vi "joint.vi"() -> ()   [LabVIEW 2023]
panel:
  out "CH2_spreadsheet":string
  out "CH2_array_units":dbl[][](array[numeric])
  out "CH2_Time":dbl[](array[numeric])
  out "CH2_Voltage":dbl[](array[numeric])
  out "CH2_array":dbl[][](array[numeric])
  out "concatenated string 2":string
  out "CH2_file":string
  in  "match button":bool
  in  "STOP":bool
  in  "Export button":bool
  out "CH1_spreadsheet":string
  out "CH1_array_units":dbl[][](array[numeric])
  out "CH1_Time":dbl[](array[numeric])
  out "CH1_Voltage":dbl[](array[numeric])
  out "CH1_file":string
  in  "index":i32 min=0 max=20
  out "CH1_array":dbl[][](array[numeric])
  out "concatenated string":string
  in  "R (Ω)":string
  in  "Current mode":bool
  in  "Extract button":bool
  out "standard output":string
  in  "CH2_units":string(combo)
  in  "∆V CH2":string
  in  "CH1_units":string(combo)
  in  "∆V CH1":string
  in  "t units":string(combo)
  in  "∆t":string
  out "CH1":bool
  out "CH2":bool
  in  "Select channel":bool
  in  "Output path":path
  in  "Input path":path
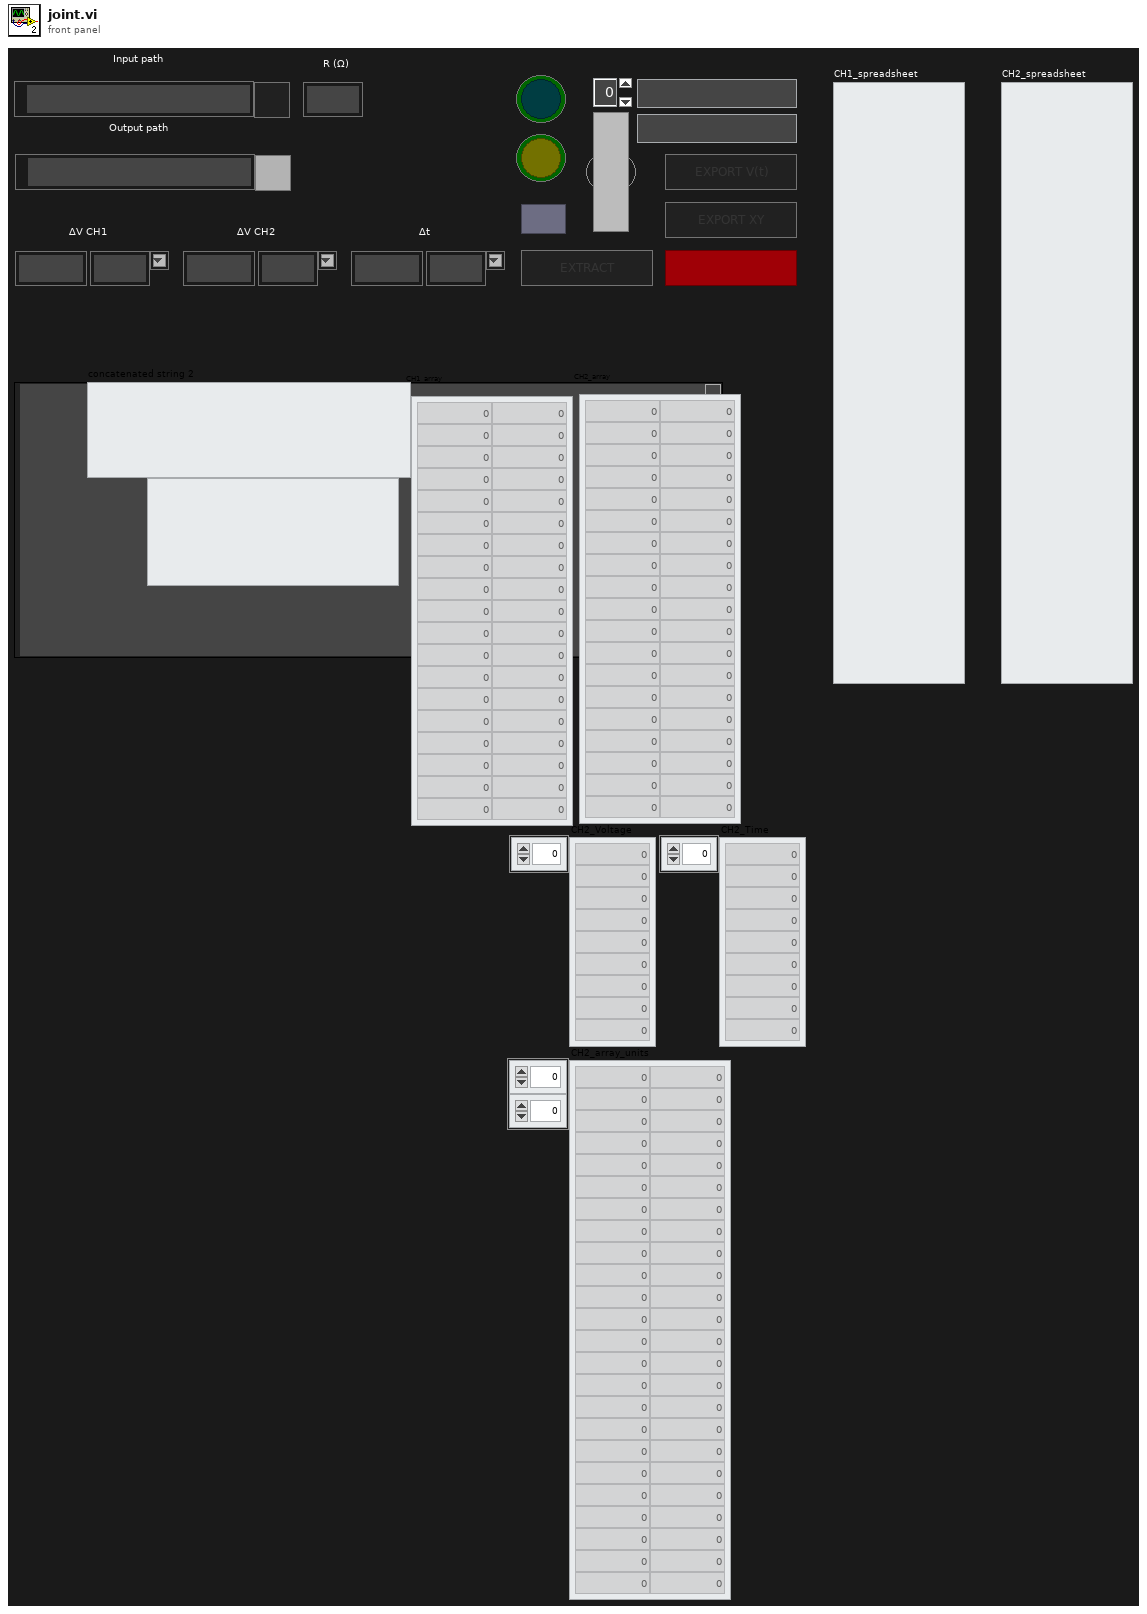
[diagram p1: front panel]
types:
  T1 = enum16{"open", "replace", "create", "open or create", "replace or create", "replace or create with confirmation"}
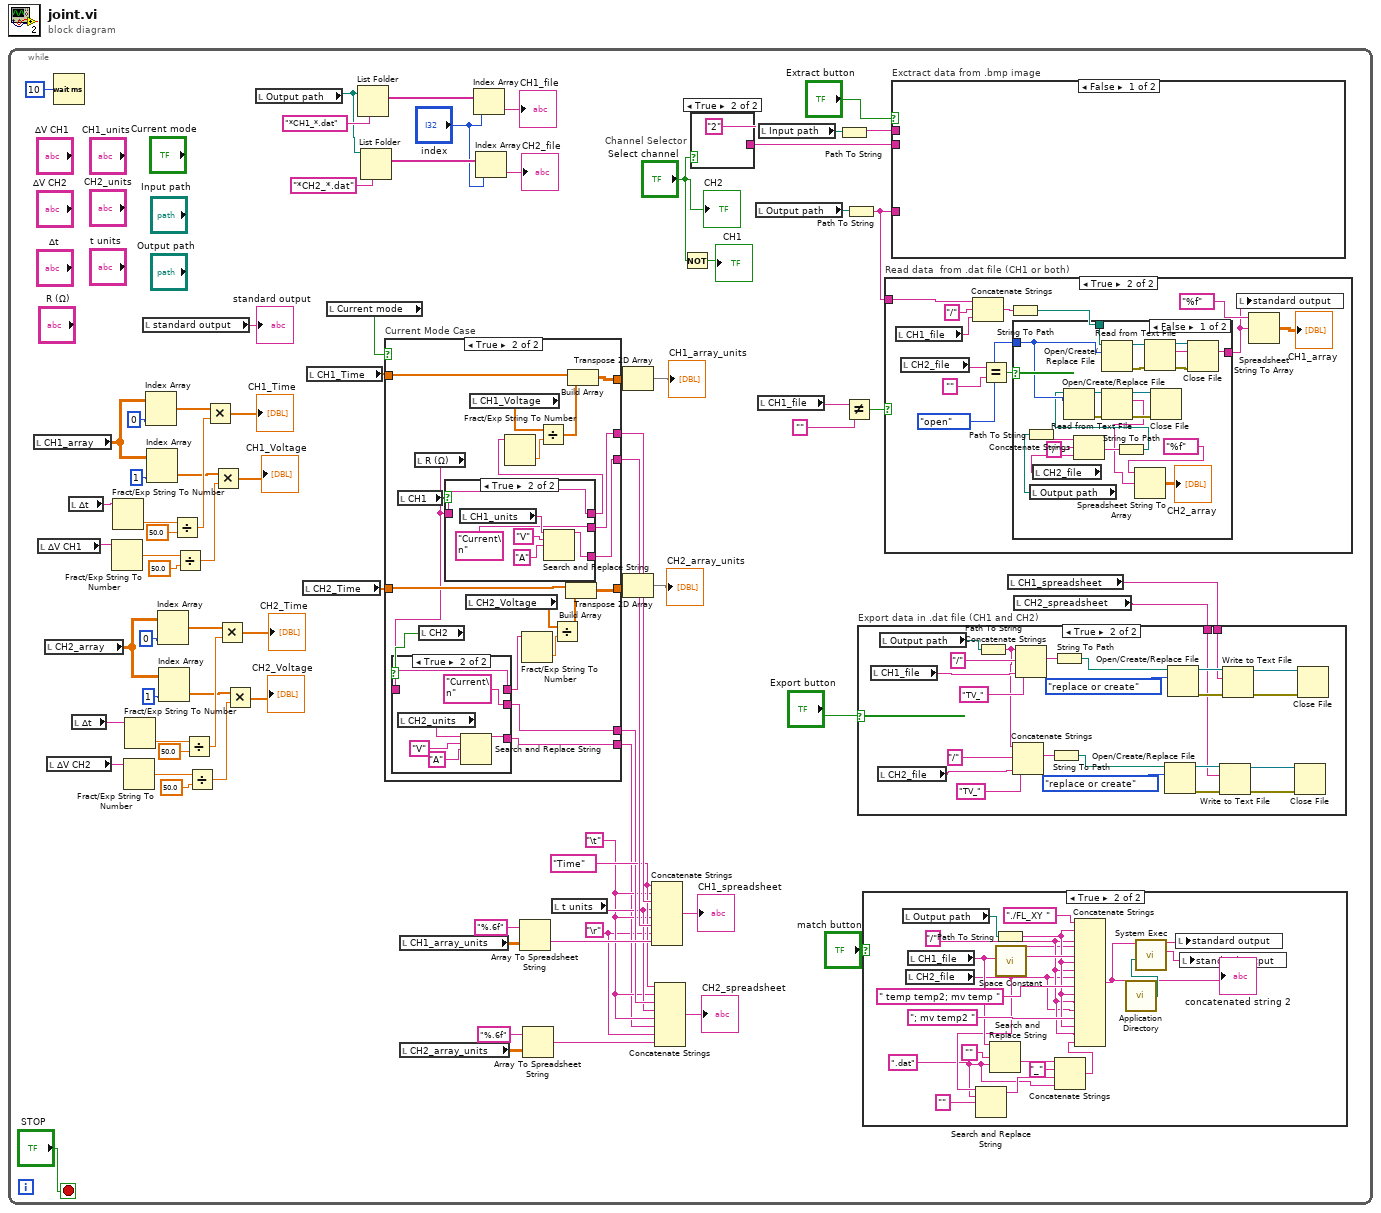
[diagram p0: block diagram]
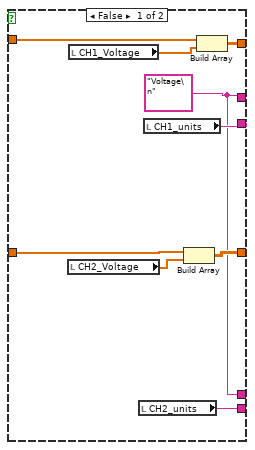
[diagram p2: hidden frame]
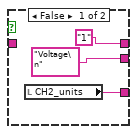
[diagram p3: hidden frame]
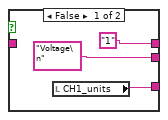
[diagram p4: hidden frame]
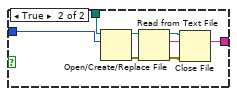
[diagram p8: hidden frame]
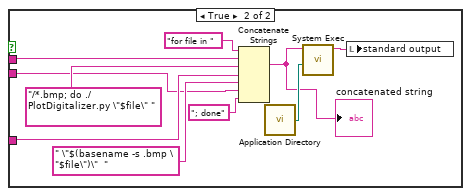
[diagram p9: hidden frame]
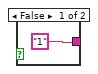
[diagram p10: hidden frame]
diagram:
  n1 = while {
    stop <- "STOP" stop-if-true
    w4 = "\r"
    w6 = "\t"
    w9 = "Time" ("string")
    n2 = local read "CH1_array"() -> (w72:dbl[][])
    n3 = local read "∆V CH1"() -> (w41:string)
    n4 = local read "CH2_array"() -> (w25:dbl[][])
    n5 = local read "∆V CH2"() -> (w23:string)
    n6 = Wait (ms)(milliseconds to wait=u32 10) -> ()  [unwired: 1 out]
    n7 = local read "∆t"() -> (w65:string)
    n8 = local read "∆t"() -> (w24:string)
    n9 = Fract/Exp String To Number(string=w41) -> (number=w66:dbl)  [unwired: 3 in, 1 out]
    n10 = Fract/Exp String To Number(string=w65) -> (number=w63:dbl)  [unwired: 3 in, 1 out]
    n11 = Fract/Exp String To Number(string=w23) -> (number=w34:dbl)  [unwired: 3 in, 1 out]
    n12 = Fract/Exp String To Number(string=w24) -> (number=w32:dbl)  [unwired: 3 in, 1 out]
    n13 = local read "standard output"() -> (→"standard output":string)
    n14 = Index Array(array=w72, index (col)=0 ("disabled index (col)")) -> (element=w43:dbl[])  [unwired: 1 in]
    n15 = Index Array(array=w72, index (col)=1 ("disabled index (col)")) -> (element=w40:dbl[])  [unwired: 1 in]
    n16 = Index Array(array=w25, index (col)=0 ("disabled index (col)")) -> (element=w30:dbl[])  [unwired: 1 in]
    n17 = Index Array(array=w25, index (col)=1 ("disabled index (col)")) -> (element=w28:dbl[])  [unwired: 1 in]
    n18 = Divide(x=w63, y=50.0) -> (x/y=w42:dbl)
    n19 = Divide(x=w66, y=50.0) -> (x/y=w39:dbl)
    n20 = Divide(x=w32, y=50.0) -> (x/y=w29:dbl)
    n21 = Divide(x=w34, y=50.0) -> (x/y=w27:dbl)
    n22 = Multiply(x=w43, y=w42) -> (x*y=→"CH1_Time":dbl[])
    n23 = Multiply(x=w40, y=w39) -> (x*y=→"CH1_Voltage":dbl[])
    n24 = Multiply(x=w30, y=w29) -> (x*y=→"CH2_Time":dbl[])
    n25 = Multiply(x=w28, y=w27) -> (x*y=→"CH2_Voltage":dbl[])
    n26 = local read "Output path"() -> (w45:path)
    n27 = local read "CH2_Time"() -> (w20:dbl[])
    n28 = local read "CH1_Time"() -> (w21:dbl[])
    n29 = local read "Current mode"() -> (w22:bool)
    n30 = List Folder(path=w45, pattern="*CH1_*.dat") -> (filenames=w69:string[])  [unwired: 2 in, 3 out]
    n31 = List Folder(path=w45, pattern="*CH2_*.dat") -> (filenames=w54:string[])  [unwired: 2 in, 3 out]
    n32 = case "Current Mode Case" shown="True" w22 {
      tunnel: [w87 w107] -> w61
      tunnel: w21 -> [w88 w105]
      tunnel: w20 -> [w85 w104]
      tunnel: [w83 w106] -> w18
      tunnel: [w81 w91] -> w15
      tunnel: [w82 w92] -> w14
      tunnel: [w81 w90] -> w8
      tunnel: [w80 w89] -> w5
      frame False {
        w81 = "Voltage\n"
        n33 = local read "CH2_Voltage"() -> (w84:dbl[])
        n34 = local read "CH1_Voltage"() -> (w86:dbl[])
        n35 = local read "CH2_units"() -> (w80:string)
        n36 = local read "CH1_units"() -> (w82:string)
        n37 = Build Array(w85, w84) -> (w83:dbl[][])
        n38 = Build Array(w88, w86) -> (w87:dbl[][])
      }
      frame True {
        n39 = local read "CH1"() -> (w96:bool)
        n40 = local read "R (Ω)"() -> (w93:string)
        n41 = local read "CH2"() -> (w94:bool)
        n42 = case shown="True" w94 {
          tunnel: w93 -> [_ w116]
          tunnel: ["1" w116] -> w95
          tunnel: ["Voltage\n" "Current\n"] -> w90
          tunnel: [w108 w113] -> w89
          frame False {
            n43 = local read "CH2_units"() -> (w108:string)
          }
          frame True {
            n44 = local read "CH2_units"() -> (w111:string)
            n45 = Search and Replace String(input string=w111, search string="V", replace string="A") -> (result string=w113:string)  [unwired: 5 in, 3 out]
          }
        }
        n46 = case shown="True" w96 {
          tunnel: w93 -> [_ w125]
          tunnel: ["1" w125] -> w97
          tunnel: [w118 w124] -> w92
          tunnel: ["Voltage\n" "Current\n"] -> w91
          frame False {
            n47 = local read "CH1_units"() -> (w118:string)
          }
          frame True {
            n48 = local read "CH1_units"() -> (w121:string)
            n49 = Search and Replace String(input string=w121, search string="V", replace string="A") -> (result string=w124:string)  [unwired: 5 in, 3 out]
          }
        }
        n50 = local read "CH2_Voltage"() -> (w98:dbl[])
        n51 = local read "CH1_Voltage"() -> (w103:dbl[])
        n52 = Fract/Exp String To Number(string=w97) -> (number=w101:dbl)  [unwired: 3 in, 1 out]
        n53 = Fract/Exp String To Number(string=w95) -> (number=w100:dbl)  [unwired: 3 in, 1 out]
        n54 = Divide(x=w103, y=w101) -> (x/y=w102:dbl[])
        n55 = Divide(x=w98, y=w100) -> (x/y=w99:dbl[])
        n56 = Build Array(w104, w99) -> (w106:dbl[][])
        n57 = Build Array(w105, w102) -> (w107:dbl[][])
      }
    }
    n58 = local read "CH1_array_units"() -> (w17:dbl[][])
    n59 = local read "CH2_array_units"() -> (w10:dbl[][])
    n60 = Index Array(array=w69, index="index") -> (element=→"CH1_file":string)
    n61 = Index Array(array=w54, index="index") -> (element=→"CH2_file":string)
    n62 = Array To Spreadsheet String(array=w17, 3:"%.6f" ("format string")) -> (spreadsheet string=w59:string)  [unwired: 1 in]
    n63 = Array To Spreadsheet String(array=w10, 3:"%.6f" ("format string")) -> (spreadsheet string=w3:string)  [unwired: 1 in]
    n64 = local read "t units"() -> (w7:string)
    n65 = Transpose 2D Array(2D array=w61) -> (transposed array=→"CH1_array_units":dbl[][])
    n66 = Transpose 2D Array(2D array=w18) -> (transposed array=→"CH2_array_units":dbl[][])
    n67 = Concatenate Strings(w9, w6, w15, w7, w6, w14, w4, w59) -> (→"CH1_spreadsheet":string)
    n68 = Concatenate Strings(w9, w6, w8, w7, w6, w5, w4, w3) -> (→"CH2_spreadsheet":string)
    n69 = Not(x="Select channel") -> (.not. x?=→"CH1":bool)
    n70 = case "Channel Selector" shown="True" "Select channel" {
      tunnel: ["1" "2"] -> w71
      frame False {
      }
      frame True {
      }
    }
    n71 = local read "Output path"() -> (w48:path)
    n72 = local read "CH1_file"() -> (w52:string)
    n73 = local read "Input path"() -> (w47:path)
    n74 = Path To String(path=w47) -> (string=w76:string)
    n75 = Not Equal?(x=w52, y="") -> (x != y?=w44:bool)
    n76 = Path To String(path=w48) -> (string=w46:string)
    n77 = case shown="True" "match button" {
      frame False {
      }
      frame True {
        w127 = ".dat"
        w135 = "/" ("string")
        n78 = local read "Output path"() -> (w142:path)
        n79 = local read "CH2_file"() -> (w129:string)
        n80 = local read "CH1_file"() -> (w134:string)
        n81 = Search and Replace String(input string=w129, search string=w127, replace string="" ("replace string (\"\")")) -> (result string=w128:string)  [unwired: 5 in, 3 out]
        n82 = Search and Replace String(input string=w134, search string=w127, replace string="" ("replace string (\"\")")) -> (result string=w132:string)  [unwired: 5 in, 3 out]
        n83 = Path To String(path=w142) -> (string=w136:string)
        n84 = call <vilib>:"Space Constant.vi"() -> ("String"=w138:string)
        n85 = Concatenate Strings(w132, "_" ("string"), w128, w127) -> (w126:string)
        n86 = Concatenate Strings("./FL_XY " ("string"), w136, w135, w134, w138, w136, w135, w129, " temp temp2; mv temp " ("string"), w136, w135, w129, "; mv temp2 " ("string"), w136, w135, w126) -> (w140:string)
        "concatenated string 2" <- w140
        n87 = call <vilib>:"Application Directory.vi"() -> ("Application Directory"=w145:path)
        n88 = call <vilib>:"System Exec.vi"("working directory"=w145, "command line"=w140) -> ("standard error"=w139:string, "standard output"=w144:string)  [unwired: 6 in, 2 out]
        n89 = local write "standard output"(w144) -> ()
        n90 = local write "standard output"(w139) -> ()
      }
    }
    n91 = case "Read data  from .dat file (CH1 or both)" shown="True" w44 {
      tunnel: w46 -> [_ w173]
      frame False {
      }
      frame True {
        n92 = local read "CH1_file"() -> (w179:string)
        n93 = local read "CH2_file"() -> (w171:string)
        n94 = Concatenate Strings(w173, "/" ("string"), w179) -> (w177:string)
        n95 = Equal?(x=w171, y="") -> (x = y?=w172:bool)
        n96 = String To Path(string=w177) -> (path=w178:path)
        n97 = case shown="False" w172 {
          tunnel: w178 -> [w199 w206]
          tunnel: T1."open" ("operation (0:open)") -> [w191 w205]
          tunnel: [w196 w202] -> w174
          frame False {
            n98 = local read "Output path"() -> (w186:path)
            n99 = Path To String(path=w186) -> (string=w187:string)
            n100 = local read "CH2_file"() -> (w185:string)
            n101 = Concatenate Strings(w187, "/" ("string"), w185) -> (w190:string)
            n102 = Open/Create/Replace File(file path (use dialog)=w199, operation (0:open)=w191) -> (refnum out=w198:refnum<file>, error out=w200:errorcluster)  [unwired: 4 in, 1 out]
            n103 = String To Path(string=w190) -> (path=w188:path)
            n104 = Open/Create/Replace File(file path (use dialog)=w188, operation (0:open)=w191) -> (refnum out=w192:refnum<file>, error out=w194:errorcluster)  [unwired: 4 in, 1 out]
            n105 = Read from Text File(file (use dialog)=w192, error in=w194) -> (refnum out=w193:refnum<file>, text=w183:string, error out=w195:errorcluster)  [unwired: 2 in, 1 out]
            n106 = Spreadsheet String To Array(format string="%f", spreadsheet string=w183) -> (array=→"CH2_array":dbl[][])  [unwired: 2 in]
            n107 = Read from Text File(file (use dialog)=w198, error in=w200) -> (refnum out=w197:refnum<file>, text=w196:string, error out=w201:errorcluster)  [unwired: 2 in, 1 out]
            n108 = Close File(refnum=w193, error in=w195) -> ()  [unwired: 2 out]
            n109 = Close File(refnum=w197, error in=w201) -> ()  [unwired: 2 out]
          }
          frame True {
            n110 = Open/Create/Replace File(file path (use dialog)=w206, operation (0:open)=w205) -> (refnum out=w204:refnum<file>, error out=w203:errorcluster)  [unwired: 4 in, 1 out]
            n111 = Read from Text File(file (use dialog)=w204, error in=w203) -> (refnum out=w207:refnum<file>, text=w202:string, error out=w208:errorcluster)  [unwired: 2 in, 1 out]
            n112 = Close File(refnum=w207, error in=w208) -> ()  [unwired: 2 out]
          }
        }
        n113 = local write "standard output"(w174) -> ()
        n114 = Spreadsheet String To Array(format string="%f", spreadsheet string=w174) -> (array=→"CH1_array":dbl[][])  [unwired: 2 in]
      }
    }
    n115 = case "Exctract data from .bmp image" shown="False" "Extract button" {
      tunnel: w76 -> [_ w215]
      tunnel: w71 -> [_ w209]
      tunnel: w46 -> [_ w212]
      frame False {
      }
      frame True {
        n116 = Concatenate Strings("for file in ", w215, "/*.bmp; do ./PlotDigitalizer.py \"$file\" " ("string"), w212, " \"$(basename -s .bmp \"$file\")\"  " ("string"), w209, "; done" ("string")) -> (w214:string)
        "concatenated string" <- w214
        n117 = call <vilib>:"Application Directory.vi"() -> ("Application Directory"=w217:path)
        n118 = call <vilib>:"System Exec.vi"("working directory"=w217, "command line"=w214) -> ("standard output"=w218:string)  [unwired: 6 in, 3 out]
        n119 = local write "standard output"(w218) -> ()
      }
    }
    n120 = local read "CH1_spreadsheet"() -> (w13:string)
    n121 = local read "CH2_spreadsheet"() -> (w1:string)
    n122 = case "Export data in .dat file (CH1 and CH2)" shown="True" "Export button" {
      tunnel: w13 -> [_ w158]
      tunnel: w1 -> [_ w148]
      frame False {
      }
      frame True {
        n123 = local read "CH1_file"() -> (w164:string)
        n124 = local read "CH2_file"() -> (w147:string)
        n125 = local read "Output path"() -> (w163:path)
        n126 = Path To String(path=w163) -> (string=w146:string)
        n127 = Concatenate Strings(w146, "/" ("string"), "TV_" ("string"), w147) -> (w149:string)
        n128 = Concatenate Strings(w146, "/" ("string"), "TV_" ("string"), w164) -> (w159:string)
        n129 = String To Path(string=w149) -> (path=w150:path)
        n130 = String To Path(string=w159) -> (path=w160:path)
        n131 = Open/Create/Replace File(file path (use dialog)=w150, operation (0:open)=T1."replace or create") -> (refnum out=w156:refnum<file>, error out=w153:errorcluster)  [unwired: 4 in, 1 out]
        n132 = Open/Create/Replace File(file path (use dialog)=w160, operation (0:open)=T1."replace or create") -> (refnum out=w168:refnum<file>, error out=w165:errorcluster)  [unwired: 4 in, 1 out]
        n133 = Write to Text File(file (use dialog)=w156, text=w148, error in=w153) -> (refnum out=w155:refnum<file>, error out=w154:errorcluster)  [unwired: 1 in, 1 out]
        n134 = Write to Text File(file (use dialog)=w168, text=w158, error in=w165) -> (refnum out=w167:refnum<file>, error out=w166:errorcluster)  [unwired: 1 in, 1 out]
        n135 = Close File(refnum=w155, error in=w154) -> ()  [unwired: 2 out]
        n136 = Close File(refnum=w167, error in=w166) -> ()  [unwired: 2 out]
      }
    }
    "CH2" <- "Select channel"
  }
